vi "CONVERT BYU ICN DATA.vi"(11 "BYU ICN DATA IN":T1) -> (3 "ITEM DATA OUT":T2)   [LabVIEW 2019]
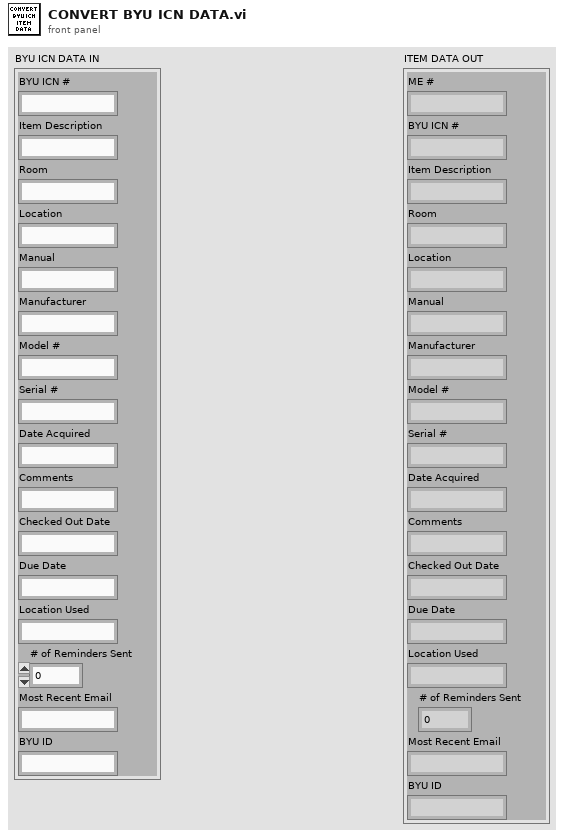
[diagram p1: front panel]
types:
  T1 = cluster{"BYU ICN #":string, "Item Description":string, "Room":string, "Location":string, "Manual":string, "Manufacturer":string, "Model #":string, "Serial #":string, "Date Acquired":string, "Comments":string, "Checked Out Date":string, "Due Date":string, "Location Used":string, "# of Reminders Sent":i32, "Most Recent Email":string, "BYU ID":string}
  T2 = cluster{"ME #":string, "BYU ICN #":string, "Item Description":string, "Room":string, "Location":string, "Manual":string, "Manufacturer":string, "Model #":string, "Serial #":string, "Date Acquired":string, "Comments":string, "Checked Out Date":string, "Due Date":string, "Location Used":string, "# of Reminders Sent":i32, "Most Recent Email":string, "BYU ID":string}
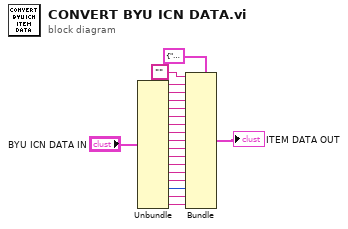
[diagram p0: block diagram]
diagram:
  n1 = Unbundle("BYU ICN DATA IN") -> ("BYU ICN #"=w15:string, "Item Description"=w14:string, "Room"=w13:string, "Location"=w11:string, "Manual"=w12:string, "Manufacturer"=w9:string, "Model #"=w10:string, "Serial #"=w8:string, "Date Acquired"=w5:string, "Comments"=w7:string, "Checked Out Date"=w4:string, "Due Date"=w6:string, "Location Used"=w3:string, "# of Reminders Sent"=w2:i32, "Most Recent Email"=w1:string, "BYU ID"=w16:string)
  n2 = Bundle(cluster=T2 {"ME #"="", "BYU ICN #"="", "Item Description"="", "Room"="", "Location"="", "Manual"="", "Manufacturer"="", "Model #"="", "Serial #"="", "Date Acquired"="", "Comments"="", "Checked Out Date"="", "Due Date"="", "Location Used"="", "# of Reminders Sent"=0, "Most Recent Email"="", "BYU ID"=""} ("ITEM DATA"), "ME #"="", "BYU ICN #"=w15, "Item Description"=w14, "Room"=w13, "Location"=w11, "Manual"=w12, "Manufacturer"=w9, "Model #"=w10, "Serial #"=w8, "Date Acquired"=w5, "Comments"=w7, "Checked Out Date"=w4, "Due Date"=w6, "Location Used"=w3, "# of Reminders Sent"=w2, "Most Recent Email"=w1, "BYU ID"=w16) -> (→"ITEM DATA OUT":T2)
